vi "FTW-TestStep-Wait-Core_Step.vi"(0 "FTW Actor Instance Configuration":string="{\n  \"Identity\": \"Wait\",\n  \"InboxAddress\": \"inproc://*\",\n  \"LoggerAddress\": \"\",\n  \"Wait Time\": 1\n}", 11 "ErrorIn":errorcluster) -> (15 "Error":errorcluster)   [LabVIEW 2015, in "FTW-TestStep-Wait-Core.lvclass"]
uses:
  FTW-TestStep-Wait-Core.lvclass
  FTW-TestStep-Wait-Core.lvclass/FTW-TestStep-Wait-Core.ctl
  source/actor/Instance/FTW-ActorInstance.lvclass/FTW-ActorInstance.ctl
  source/actor/JobSequencer/FTW-SEQ-Current.vi
  source/actor/Message/Base/FTW-Message.lvclass
  source/actor/Instance/FTW-ActorInstance.lvclass
  source/actor/Message/Request/FTW-Message-IncomingRequest.lvclass
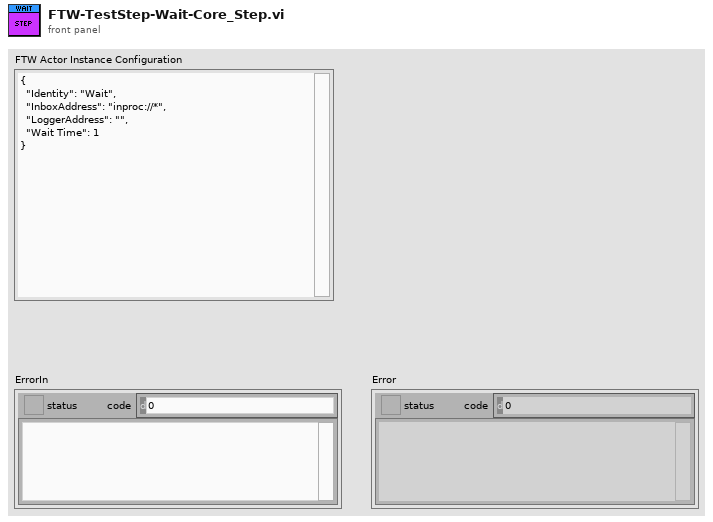
[diagram p1: front panel]
types:
  T1 = cluster{"Incoming Requests":refnum<event-registration>, "Local Messages":refnum<event-registration>, "Subscriber Registration":refnum<event-registration>}
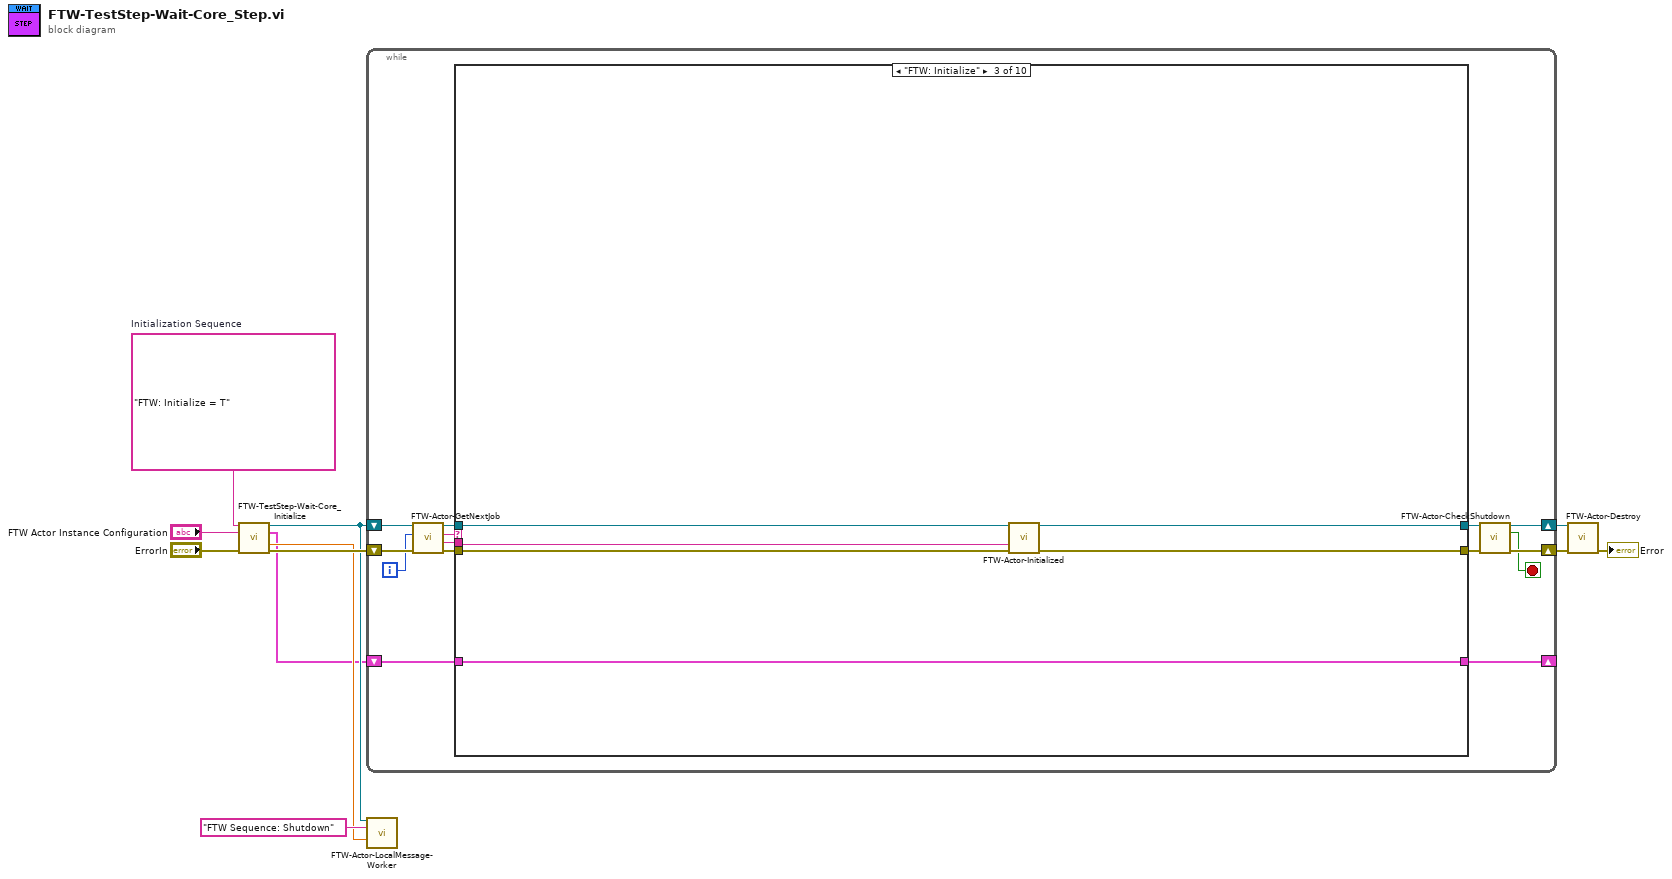
[diagram p0: block diagram]
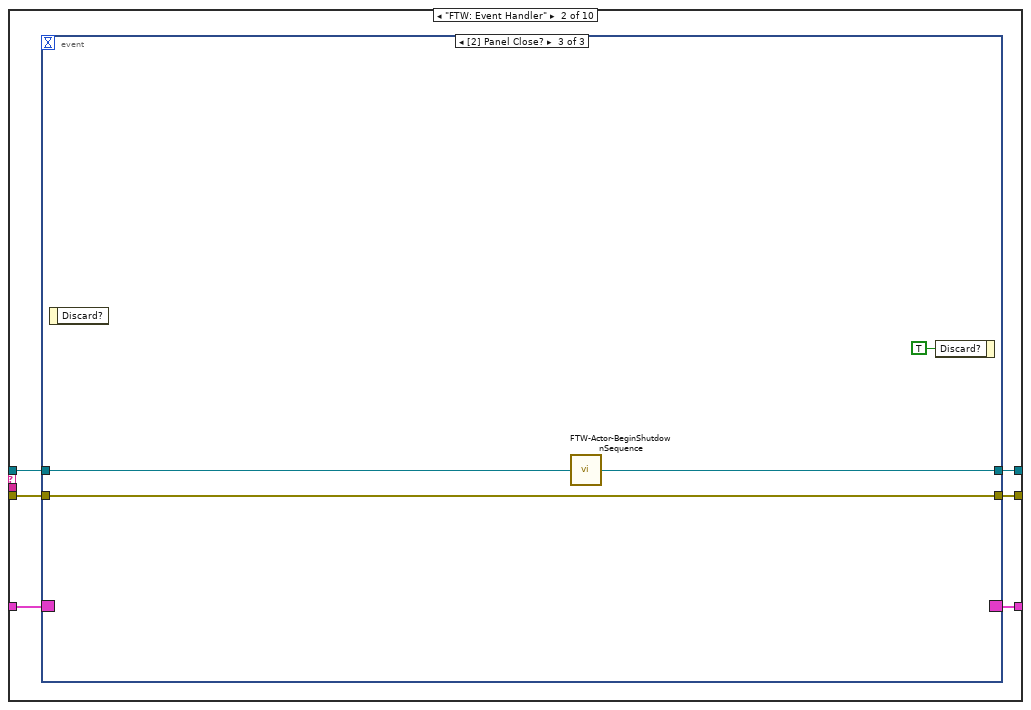
[diagram p3: hidden frame]
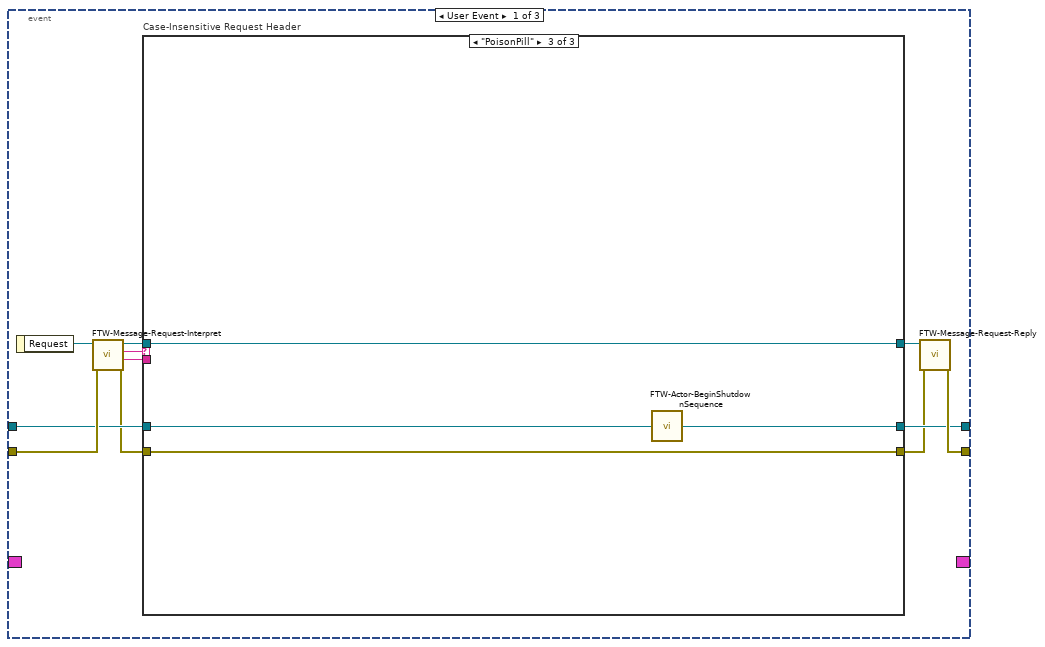
[diagram p4: hidden frame]
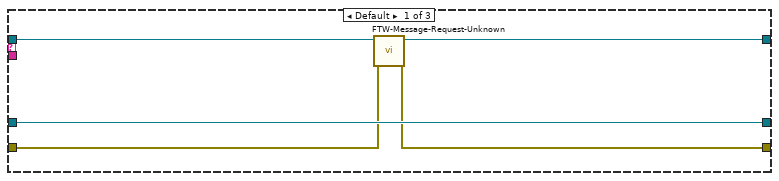
[diagram p5: hidden frame]
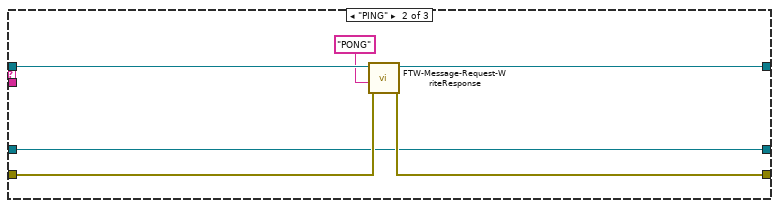
[diagram p6: hidden frame]
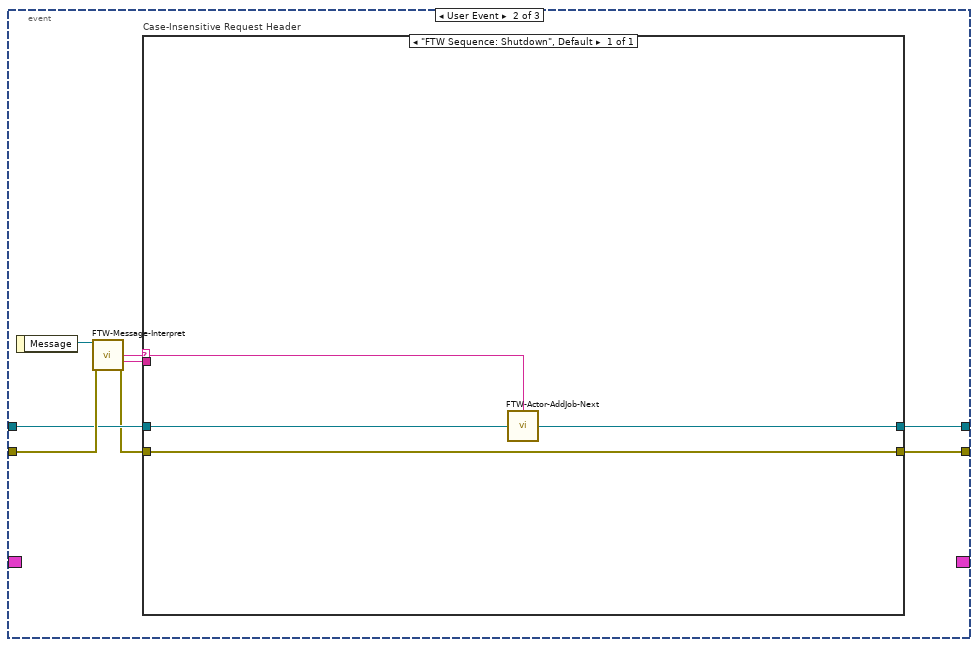
[diagram p7: hidden frame]
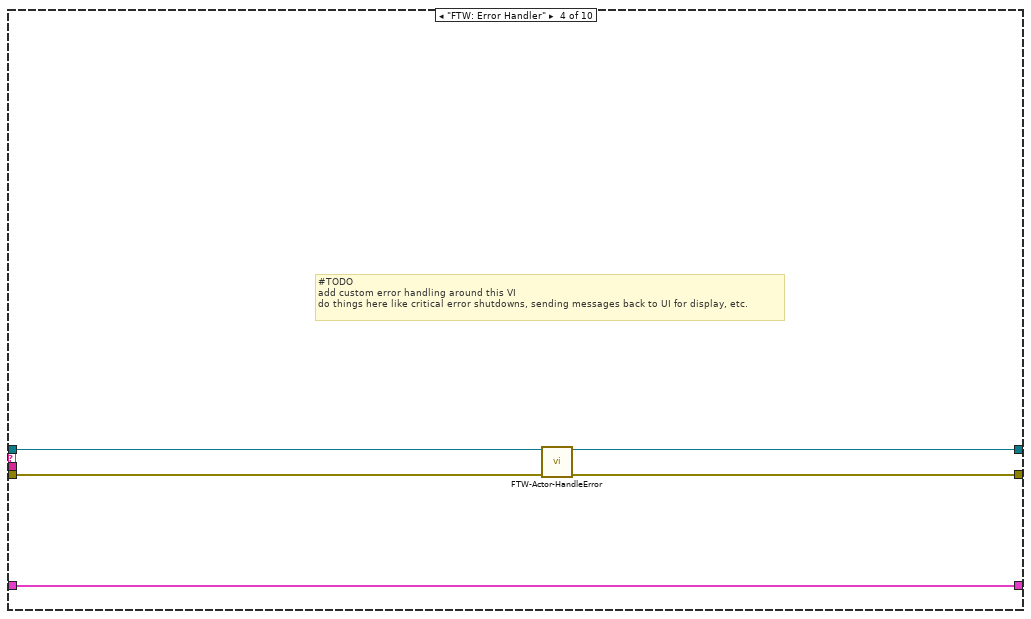
[diagram p8: hidden frame]
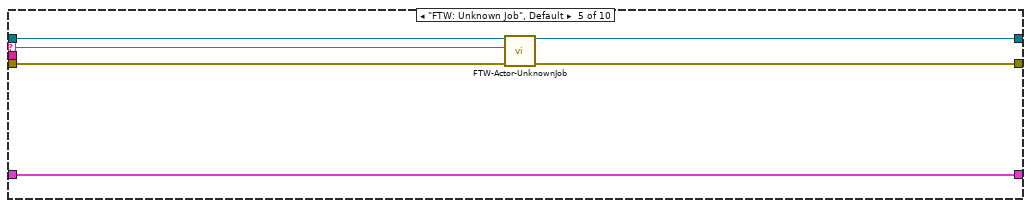
[diagram p9: hidden frame]
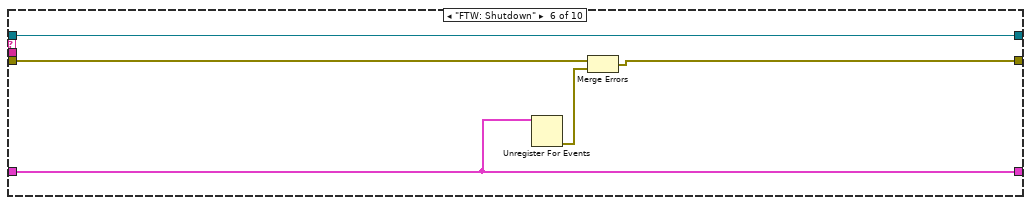
[diagram p10: hidden frame]
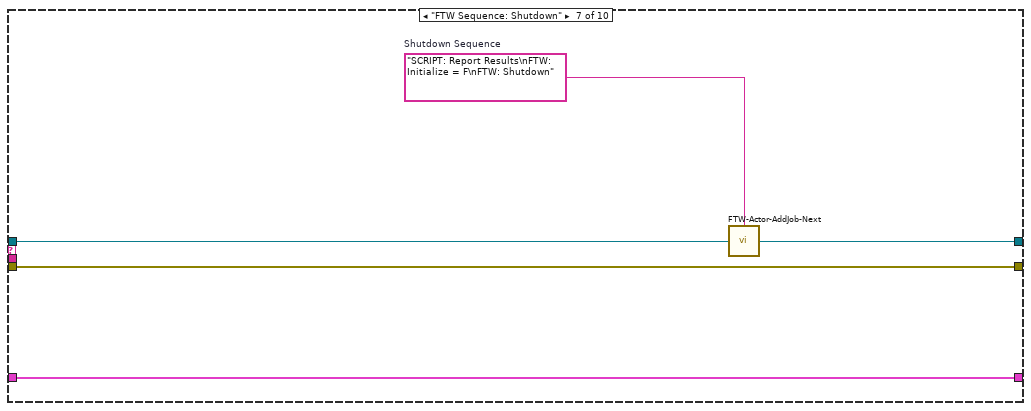
[diagram p11: hidden frame]
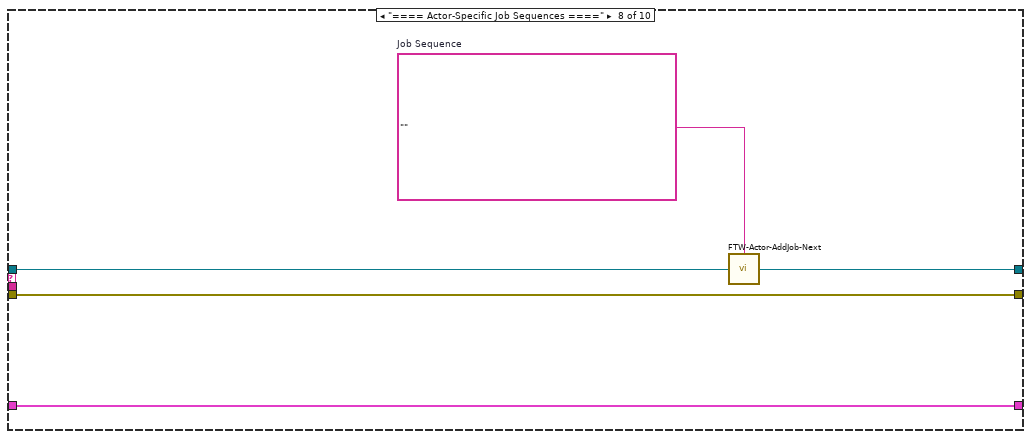
[diagram p12: hidden frame]
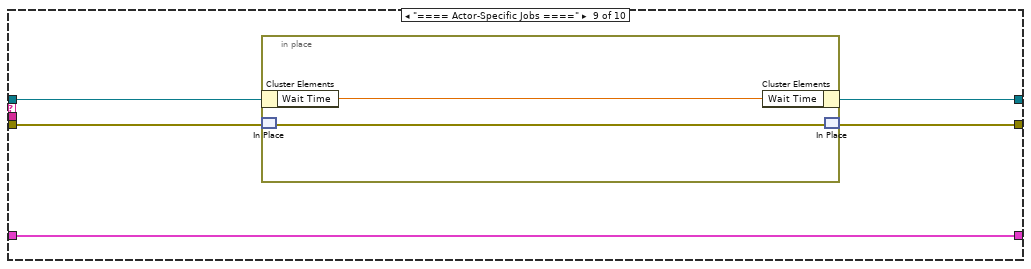
[diagram p13: hidden frame]
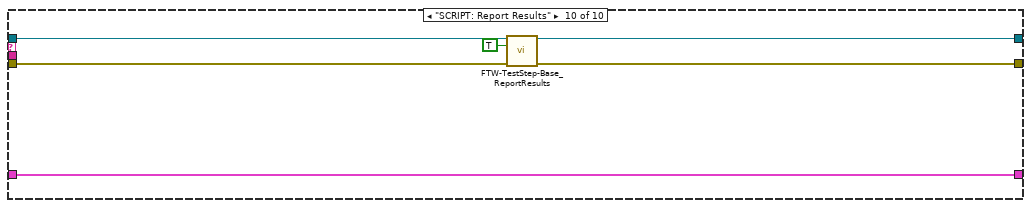
[diagram p14: hidden frame]
diagram:
  w7 = "FTW: Initialize = T"  # Initialization Sequence
  n1 = call "FTW-TestStep-Wait-Core_Initialize.vi"("Initialization Sequence"=w7, "FTW Actor Instance Configuration"="FTW Actor Instance Configuration", "error in (no error)"="ErrorIn") -> ("FTW-ScripterStep-Wait-Core Out"=w3:refnum<class "FTW-TestStep-Wait-Core.lvclass">, "Event Refnums"=w1:T1, "Wait Time"=w2:dbl, "error out"=w8:errorcluster)  [unwired: 9 in]
  n2 = while {
    shift-right: [w15] -> w10
    shift-left: w8 -> [w22]
    shift-right: [w12] -> _
    shift-left: w1 -> [w25]
    shift-right: [w17] -> w11
    shift-left: w3 -> [w24]
    i -> [w13]
    stop <- w14 stop-if-true
    n3 = call "FTW-Actor-GetNextJob.vi"("error in"=w22, "Jobs Performed"=w13, "FTW Actor Instance"=w24) -> ("error out"=w21:errorcluster, "Job Data"=w19:string, "Job Name"=w20:string, "FTW Actor Instance out"=w23:refnum<class "FTW-TestStep-Wait-Core.lvclass">)  [unwired: 5 in]
    n4 = case shown="\"FTW: Initialize\"" w20 {
      selector: w20 -> [_ _ _ _ w88 _ _ _ _ _]
      tunnel: [w27 w34 w80 w83 w91 w97 w102 w107 w111 w117] -> w16
      tunnel: w21 -> [w27 w33 w77 w85 w92 w98 w102 w107 w112 w120]
      tunnel: w25 -> [w28 w29 w82 w87 w93 w95 w103 w108 w113 w121]
      tunnel: [w28 w32 w82 w87 w93 w95 w103 w108 w113 w121] -> w12
      tunnel: w19 -> [_ _ w78 _ _ _ _ _ _ _]
      tunnel: [w26 w31 w81 w84 w89 w94 w100 w105 w109 w118] -> w18
      tunnel: w23 -> [w26 w30 w79 w86 w90 w94 w101 w106 w110 w119]
      frame "==== Featherweight Framework Jobs ====" {
      }
      frame "FTW: Event Handler" {
        n5 = event shown="[2] Panel Close?" {
          selector: w29 -> [_ _ _]
          dyn-events: [_ _ _] -> w32
          timeout: _ -> [_ _ _]
          tunnel: [w44 w63 w75] -> w34
          tunnel: w33 -> [w43 w67 w75]
          tunnel: [w38 w64 w73] -> w31
          tunnel: w30 -> [w42 w66 w74]
          event User Event {
            n6 = event-data() -> ("Request"=w45:refnum<class "FTW-Message-IncomingRequest.lvclass">)  [unwired: 1 in]
            n7 = call "FTW-Message-Request-Interpret.vi"("error in"=w43, "FTW Incoming Request"=w45) -> ("error out"=w41:errorcluster, "Request Body"=w35:string, "Request Header"=w39:string, "FTW Incoming Request out"=w40:refnum<class "FTW-Message-IncomingRequest.lvclass">)  [unwired: 6 in]
            n8 = case "Case-Insensitive Request Header" shown="\"PoisonPill\"" w39 {
              tunnel: [w48 w54 w59] -> w37
              tunnel: w41 -> [w49 w55 w59]
              tunnel: [w50 w53 w60] -> w38
              tunnel: w42 -> [w50 w53 w58]
              tunnel: w40 -> [w47 w56 w57]
              tunnel: [w46 w52 w57] -> w36
              tunnel: w35 -> [_ _ _]
              frame Default {
                n9 = call "FTW-Message-Request-Unknown.vi"("error in"=w49, "FTW Incoming Request"=w47) -> ("error out"=w48:errorcluster, "FTW Incoming Request Out"=w46:refnum<class "FTW-Message-IncomingRequest.lvclass">)  [unwired: 8 in]
              }
              frame "PING" {
                n10 = call "FTW-Message-Request-WriteResponse.vi"("error in"=w55, "Response Body"="PONG" ("Response Header"), "FTW Incoming Request"=w56) -> ("error out"=w54:errorcluster, "FTW Incoming Request out"=w52:refnum<class "FTW-Message-IncomingRequest.lvclass">)  [unwired: 7 in]
              }
              frame "PoisonPill" {
                n11 = call "FTW-Actor-BeginShutdownSequence.vi"("FTW Actor Instance"=w58) -> ("FTW Actor Instance out"=w60:refnum<class "FTW-TestStep-Wait-Core.lvclass">)  [unwired: 3 in]
              }
            }
            n12 = call "FTW-Message-Request-Reply.vi"("FTW: Reply Error"=w37, "FTW Incoming Request"=w36) -> ("error out"=w44:errorcluster)  [unwired: 8 in, 1 out]
          }
          event User Event {
            n13 = event-data() -> ("Message"=w68:refnum<class "FTW-Message.lvclass">)  [unwired: 1 in]
            n14 = call-dynamic "FTW-Message-Interpret.vi"("FTW Message"=w68, "error in"=w67) -> ("Message Header"=w62:string, "Message Body"=w61:string, "error out"=w65:errorcluster)  [unwired: 9 in, 2 out]
            n15 = case "Case-Insensitive Request Header" shown="\"FTW Sequence: Shutdown\", Default" w62 {
              selector: w62 -> [w69]
              tunnel: [w71] -> w63
              tunnel: w65 -> [w71]
              tunnel: [w70] -> w64
              tunnel: w66 -> [w72]
              tunnel: w61 -> [_]
              frame "FTW Sequence: Shutdown", Default {
                n16 = call "FTW-Actor-AddJob-Next.vi"("Add Next in Job Queue"=w69, "FTW Actor Instance"=w72) -> ("FTW Actor Instance out"=w70:refnum<class "FTW-TestStep-Wait-Core.lvclass">)  [unwired: 2 in]
              }
            }
          }
          event Panel Close? {
            n17 = event-data() -> ()  [unwired: 1 in, 1 out]
            n18 = call "FTW-Actor-BeginShutdownSequence.vi"("FTW Actor Instance"=w74) -> ("FTW Actor Instance out"=w73:refnum<class "FTW-TestStep-Wait-Core.lvclass">)  [unwired: 3 in]
            n19 = event-data("Discard?"=TRUE) -> ()  [unwired: 1 in, 1 out]
          }
        }
      }
      frame "FTW: Initialize" {
        n20 = call-dynamic "FTW-Actor-Initialized.vi"("FTW Actor Instance"=w79, "Positive Init?"=w78, "error in"=w77) -> ("FTW Actor Instance out"=w81:refnum<class "FTW-TestStep-Wait-Core.lvclass">, "error out"=w80:errorcluster)  [unwired: 11 in]
      }
      frame "FTW: Error Handler" {
        # "#TODO\nadd custom error handling around this VI\ndo things here like critical error shutdowns, sending messages back to UI for display, etc."
        n21 = call-dynamic "FTW-Actor-HandleError.vi"("FTW Actor Instance"=w86, "error in"=w85) -> ("FTW Actor Instance out"=w84:refnum<class "FTW-TestStep-Wait-Core.lvclass">, "error out"=w83:errorcluster)  [unwired: 10 in, 2 out]
      }
      frame "FTW: Unknown Job", Default {
        n22 = call-dynamic "FTW-Actor-UnknownJob.vi"("FTW Actor Instance"=w90, "Unknown Job"=w88, "error in"=w92) -> ("FTW Actor Instance out"=w89:refnum<class "FTW-TestStep-Wait-Core.lvclass">, "error out"=w91:errorcluster)  [unwired: 11 in]
      }
      frame "FTW: Shutdown" {
        n23 = Unregister For Events(event registration refnum=w95) -> (error out=w96:errorcluster)  [unwired: 1 in]
        n24 = Merge Errors(w98, w96) -> (w97:errorcluster)
      }
      frame "FTW Sequence: Shutdown" {
        w99 = "SCRIPT: Report Results\nFTW: Initialize = F\nFTW: Shutdown"  # Shutdown Sequence
        n25 = call "FTW-Actor-AddJob-Next.vi"("Add Next in Job Queue"=w99, "FTW Actor Instance"=w101) -> ("FTW Actor Instance out"=w100:refnum<class "FTW-TestStep-Wait-Core.lvclass">)  [unwired: 2 in]
      }
      frame "==== Actor-Specific Job Sequences ====" {
        w104 = ""  # Job Sequence
        n26 = call "FTW-Actor-AddJob-Next.vi"("Add Next in Job Queue"=w104, "FTW Actor Instance"=w106) -> ("FTW Actor Instance out"=w105:refnum<class "FTW-TestStep-Wait-Core.lvclass">)  [unwired: 2 in]
      }
      frame "==== Actor-Specific Jobs ====" {
        n27 = in-place {
          n28 = in-place-cluster #1(w110) -> ("Wait Time"=w114:dbl)
          n29 = in-place-match #2(w112) -> (w115:errorcluster)
          n30 = in-place-cluster #1("Wait Time"=w114) -> (w109:refnum<class "FTW-TestStep-Wait-Core.lvclass">)
          n31 = in-place-match #2(w115) -> (w111:errorcluster)
        }
      }
      frame "SCRIPT: Report Results" {
        n32 = call-dynamic "FTW-TestStep-Base_ReportResults.vi"("FTW-ScripterStep-Base In"=w119, "Passed"=TRUE, "error in (no error)"=w120) -> ("FTW-ScripterStep-Base Out"=w118:refnum<class "FTW-TestStep-Wait-Core.lvclass">, "error out"=w117:errorcluster)  [unwired: 11 in]
      }
    }
    n33 = call "FTW-Actor-CheckShutdown.vi"("FTW Actor Instance"=w18, "error in"=w16) -> ("FTW Actor Instance out"=w17:refnum<class "FTW-TestStep-Wait-Core.lvclass">, "Shutdown?"=w14:bool, "error out"=w15:errorcluster)  [unwired: 11 in]
  }
  n34 = call-dynamic "FTW-Actor-LocalMessage-Worker.vi"("FTW-ActorInstance In"=w3, "Message Header"="FTW Sequence: Shutdown", "Send Rate"=w2) -> ()  [unwired: 13 in]
  n35 = call-dynamic "FTW-Actor-Destroy.vi"("FTW Actor Instance"=w11, "error in"=w10) -> ("error out"=→"Error":errorcluster)  [unwired: 13 in]
